vi "GetActualDf.vi"(8 "error in":T1) -> (0 "error out":T1, 3 "Actual dF":sgl format="%#_g kHz")   [LabVIEW 2016]
doc: "Returns the current df value in mHz."
uses:
  Controls/Error_Out.ctl
  Files_ASC500/DLL/ASC500_RemoteControlV27.dll
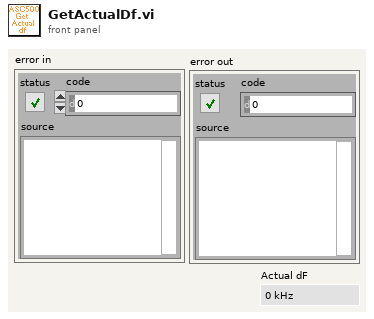
[diagram p1: front panel]
types:
  T1 = typedef "Error_Out.ctl" = errorcluster
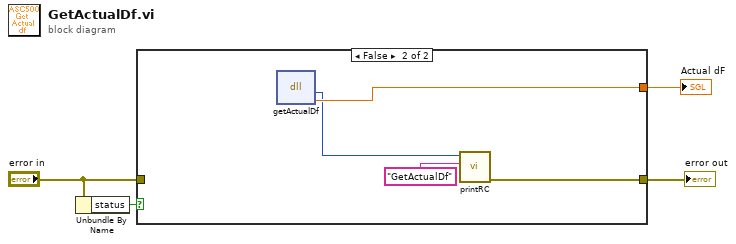
[diagram p0: block diagram]
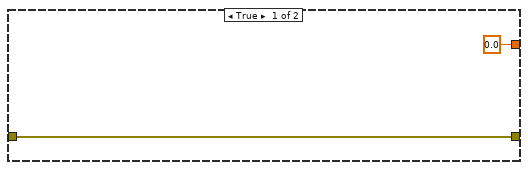
[diagram p2: hidden frame]
diagram:
  n1 = Unbundle By Name("error in") -> ("status"=w4:bool)
  n2 = case shown="False" w4 {
    tunnel: [sgl 0.0 ("Value") w10] -> w3
    tunnel: [w5 w9] -> w2
    tunnel: "error in" -> [w5 _]
    frame True {
    }
    frame False {
      n3 = dll-call lib="G:/SCMOperations/Share/ELE/Produkt Information/ASC500/04 Remote Control/02 development versions/2018Nov06/Files_ASC500/DLL/ASC500_RemoteControlV27.dll" fn="getActualDf"() -> ("return type"=w8:i32, "Value"=w10:sgl)  [unwired: 4 in, 2 out]
      n4 = call "printRC.vi"("additional information"="GetActualDf", "RC"=w8) -> ("error out"=w9:T1)  [unwired: 9 in]
    }
  }
  "error out" <- w2
  "Actual dF" <- w3
